vi "求解一元二次方程.vi"() -> ()   [LabVIEW 2018]
panel:
  out "X2":dbl
  out "X1":dbl
  in  "C":dbl
  in  "B":dbl
  in  "A":dbl
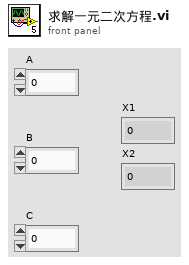
[diagram p1: front panel]
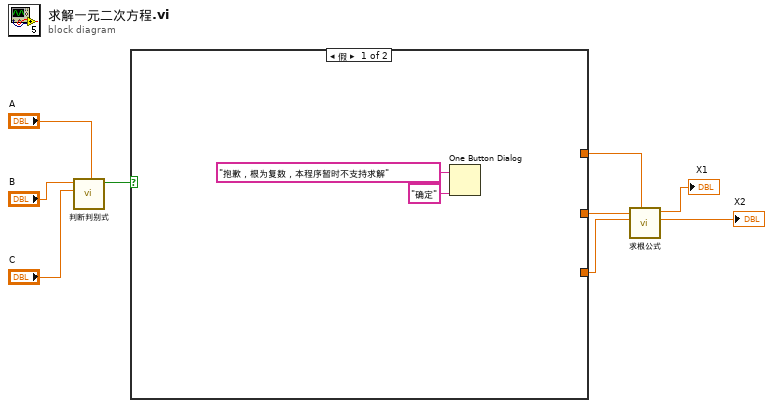
[diagram p0: block diagram]
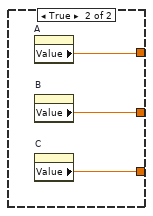
[diagram p2: hidden frame]
diagram:
  n1 = call "判断判别式.vi"("A"="A", "C"="C", "B"="B") -> ("判别式是否大于等于0"=w6:bool)  [unwired: 8 in]
  n2 = case shown="假" w6 {
    tunnel: [_ w14] -> w5
    tunnel: [_ w13] -> w4
    tunnel: [_ w12] -> w3
    frame False {
      n3 = One Button Dialog(message="抱歉，根为复数，本程序暂时不支持求解" ("消息"), button name ("OK")="确定" ("按钮名称（“确定”）")) -> ()  [unwired: 1 out]
    }
    frame True {
      n4 = property on="A" class="DigNum (严格)"() -> ("Value"=w14:dbl)  [unwired: 2 in, 2 out]
      n5 = property on="B" class="DigNum (严格)"() -> ("Value"=w13:dbl)  [unwired: 2 in, 2 out]
      n6 = property on="C" class="DigNum (严格)"() -> ("Value"=w12:dbl)  [unwired: 2 in, 2 out]
    }
  }
  n7 = call "求根公式.vi"("A"=w5, "C"=w3, "B"=w4) -> ("X2"=→"X2":dbl, "X1"=→"X1":dbl)  [unwired: 7 in]
